vi "Send Vision Data.vi"(7 "Robot IP":string, 8 "Elevator Obj Found?":bool, 9 "Elevator Obj":T1, 10 "Detected totes":T2[](array[typedef])) -> ()   [LabVIEW 2014]
uses:
  Vision Tote Data.ctl
  Common Code/Elevator Object Type.ctl
  Common Code/Vision Packet.ctl
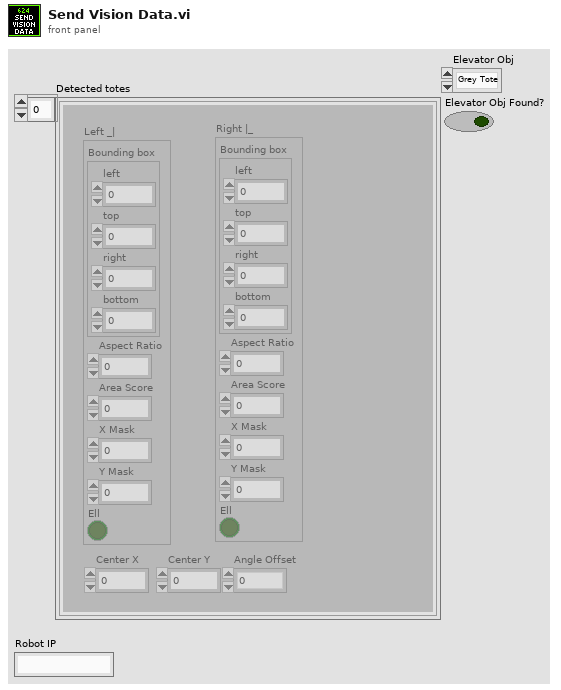
[diagram p1: front panel]
types:
  T1 = typedef "Elevator Object Type.ctl" = enum16{"Grey Tote", "Yellow Tote", "Trash Can"}
  T2 = typedef "Vision Tote Data.ctl" = cluster{"Left _|":cluster{"Bounding box":cluster{"left":dbl, "top":dbl, "right":dbl, "bottom":dbl}, "Aspect Ratio":dbl, "Area Score":dbl, "X Mask":dbl, "Y Mask":dbl, "Ell":bool}, "Right |_":cluster{"Bounding box":cluster{"left":dbl, "top":dbl, "right":dbl, "bottom":dbl}, "Aspect Ratio":dbl, "Area Score":dbl, "X Mask":dbl, "Y Mask":dbl, "Ell":bool}, "Center X":dbl, "Center Y":dbl, "Angle Offset":dbl}
  T3 = typedef "Vision Packet.ctl" = cluster{"Vision Tote":T2, "Gyro Value":dbl, "Elevator Obj Found?":bool, "Elevator Obj":T1}
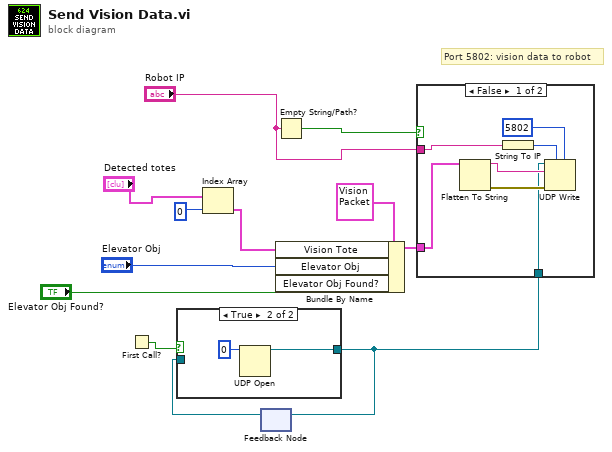
[diagram p0: block diagram]
diagram:
  # "Port 5802: vision data to robot"
  n1 = First Call?() -> (First Call?: T/F=w4:bool)
  n2 = Index Array(array="Detected totes", index=0) -> (element=w11:T2)
  n3 = feedback #1() -> (w5:refnum<k16>)  [unwired: 1 in]
  n4 = case shown="True" w4 {
    tunnel: w5 -> [w13 _]
    tunnel: [w13 w14] -> w3
    frame False {
    }
    frame True {
      n5 = UDP Open(11:u16 0 ("port")) -> (port=w14:refnum<k16>)  [unwired: 4 in, 2 out]
    }
  }
  n6 = feedback-in #1(w3) -> ()
  n7 = Empty String/Path?(string/path="Robot IP") -> (empty?=w9:bool)
  n8 = Bundle By Name(cluster=T3 {"Vision Tote"={"Left _|"={"Bounding box"={"left"=0.0, "top"=0.0, "right"=0.0, "bottom"=0.0}, "Aspect Ratio"=0.0, "Area Score"=0.0, "X Mask"=0.0, "Y Mask"=0.0, "Ell"=FALSE}, "Right |_"={"Bounding box"={"left"=0.0, "top"=0.0, "right"=0.0, "bottom"=0.0}, "Aspect Ratio"=0.0, "Area Score"=0.0, "X Mask"=0.0, "Y Mask"=0.0, "Ell"=FALSE}, "Center X"=0.0, "Center Y"=0.0, "Angle Offset"=0.0}, "Gyro Value"=0.0, "Elevator Obj Found?"=FALSE, "Elevator Obj"=enum."Grey Tote"} ("Vision Packet"), "Vision Tote"=w11, "Elevator Obj"="Elevator Obj", "Elevator Obj Found?"="Elevator Obj Found?") -> (w10:T3)
  n9 = case shown="False" w9 {
    tunnel: "Robot IP" -> [w22 _]
    tunnel: w10 -> [w21 _]
    tunnel: w3 -> [w16 _]
    frame False {
      n10 = Flatten To String(anything=w21) -> (data string=w19:string, error out=w20:errorcluster)  [unwired: 3 in, 1 out]
      n11 = String To IP(1:w22) -> (0:w18:u32)
      n12 = UDP Write(address=w18, port or service name=u16 5802, connection ID=w16, data in=w19, 8:w20) -> ()  [unwired: 1 in, 2 out]
    }
    frame True {
      # "The robot IP is not\nready yet, don't try\nto send data"
    }
  }
